vi "GetEvents.vi"(8 "error in (no error)":errorcluster, 11 "CameraDemo in":refnum<class "CameraDemo.lvclass">) -> (0 "error out":errorcluster, 2 "Events":T1, 3 "CameraDemo out":refnum<class "CameraDemo.lvclass">)   [LabVIEW 2020, in "CameraI2COUSB.lvlib" / "CameraDemo.lvclass"]
doc: "Return events generates from camera"
uses:
  CameraDemo.lvclass
  ICamera/ICamera/TypeDef/Events.ctl
  ICamera/ICamera/ICamera.lvclass
  ICamera/ICamera/TypeDef/StreamDataEvent.ctl
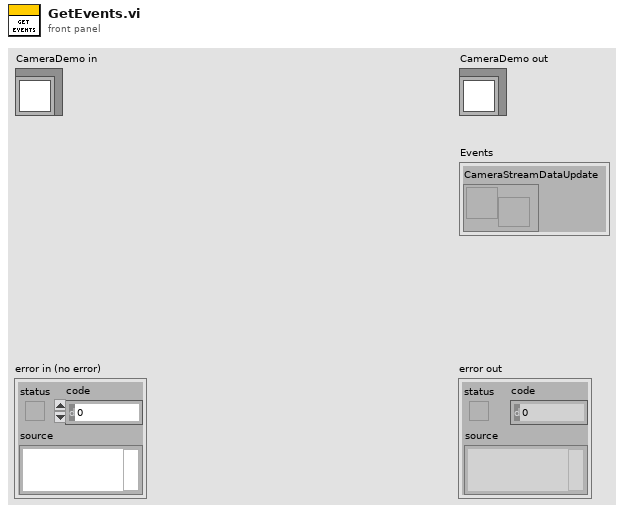
[diagram p1: front panel]
types:
  T1 = typedef "ICamera.lvlib/ICamera.lvclass/Events.ctl" = cluster{"CameraStreamDataUpdate":T2}
  T2 = typedef "ICamera.lvlib/ICamera.lvclass/StreamDataEvent.ctl" = refnum<user-event>
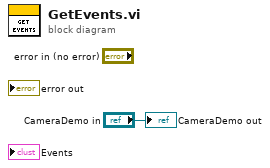
[diagram p0: block diagram]
diagram:
  "CameraDemo out" <- "CameraDemo in"
